vi "Main.vi"() -> ()   [LabVIEW 2018]
panel:
  in  "Save":bool
  in  "Data":T1={"Name"="Kevin", "Depart"="¦Û°Ê¤Æ±±¨î³¡", "Company"="¸s²Ý¯à·½ªÑ¥÷¦³­­¤½¥q", "E-Mail"="egdep33@hephasenergy.com", "Extension"="213", "Address"="·s¦Ë¿¤¶é°Ï¤G¸ô60¸¹1¼Ó"}
  in  "WebBrowser":refnum<k7>(container)
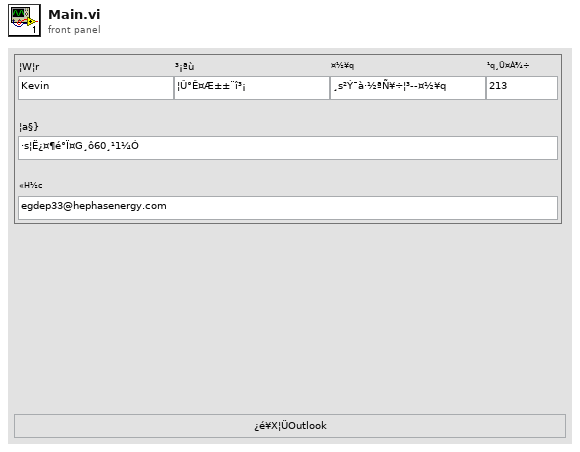
[diagram p1: front panel]
types:
  T1 = cluster{"Name":string, "Depart":string, "Company":string, "E-Mail":string, "Extension":string, "Address":string}
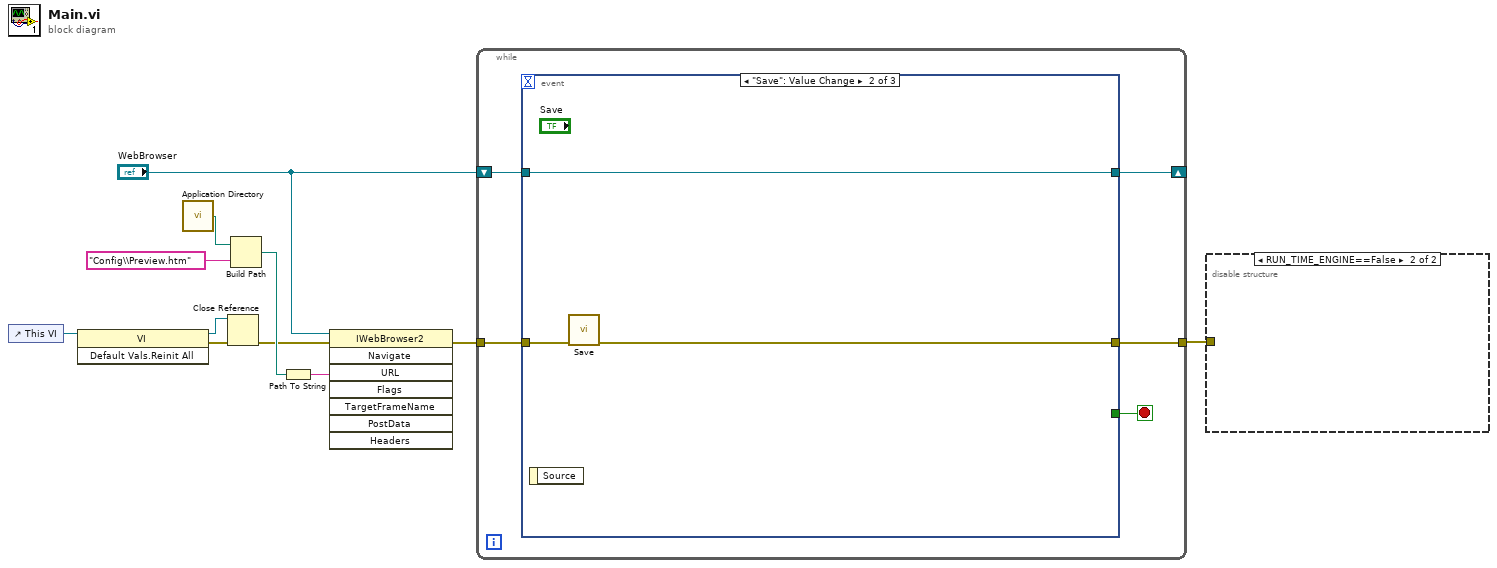
[diagram p0: block diagram]
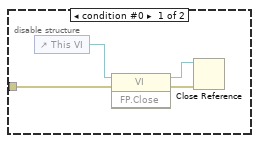
[diagram p2: hidden frame]
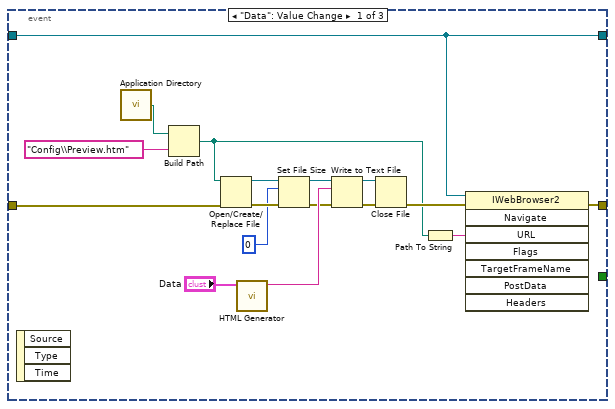
[diagram p3: hidden frame]
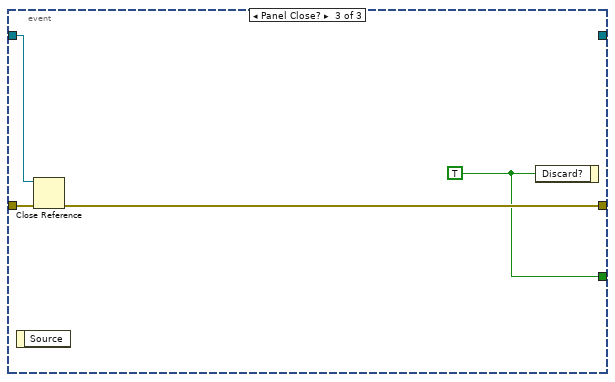
[diagram p4: hidden frame]
diagram:
  n1 = control-ref of="This VI"() -> (w5:refnum<vi>)
  n2 = invoke class="VI" method="Default Vals.Reinit All"(reference=w5) -> (reference out=w3:refnum<vi>, error out=w4:errorcluster)  [unwired: 2 in, 1 out]
  n3 = call <vilib>:"Application Directory.vi"() -> ("Application Directory"=w11:path)
  n4 = Close Reference(reference=w3, error in (no error)=w4) -> (error out=w2:errorcluster)
  n5 = Build Path(base path=w11, name or relative path="Config\\Preview.htm") -> (appended path=w8:path)
  n6 = Path To String(path=w8) -> (string=w9:string)
  n7 = invoke class="IWebBrowser2" method="Navigate"(reference="WebBrowser", error in=w2, "URL"=w9) -> (error out=w7:errorcluster)  [unwired: 5 in, 7 out]
  n8 = while {
    tunnel: w7 -> [w16]
    shift-right: [w13] -> _
    shift-left: "WebBrowser" -> [w15]
    tunnel: [w14] -> w1
    stop <- w12 stop-if-true
    n9 = event shown="[1] \"Save\": Value Change" {
      selector: _ -> [_ _ _]
      dyn-events: _ -> [_ _ _]
      timeout: _ -> [_ _ _]
      tunnel: w16 -> [w23 w35 w40]
      tunnel: w15 -> [w24 w36 w39]
      tunnel: [w25 w34 w38] -> w14
      tunnel: [w24 w36 _] -> w13
      tunnel: [_ _ w37] -> w12
      event "Data": Value Change {
        n10 = event-data() -> ()  [unwired: 1 in, 3 out]
        n11 = call <vilib>:"Application Directory.vi"() -> ("Application Directory"=w32:path)
        n12 = Build Path(base path=w32, name or relative path="Config\\Preview.htm") -> (appended path=w26:path)
        n13 = Open/Create/Replace File(file path (use dialog)=w26, error in=w23) -> (refnum out=w21:refnum<file>, error out=w20:errorcluster)  [unwired: 4 in, 1 out]
        n14 = call "HTML Generator.vi"("Data"="Data") -> ("HTML Out"=w29:string)  [unwired: 10 in]
        n15 = Set File Size(4:w20, 6:i64 0 ("size (in bytes)"), 7:w21) -> (0:w19:errorcluster, 3:w18:refnum<file>)
        n16 = Write to Text File(file (use dialog)=w18, text=w29, error in=w19) -> (refnum out=w31:refnum<file>, error out=w33:errorcluster)  [unwired: 1 in, 1 out]
        n17 = Close File(refnum=w31, error in=w33) -> (error out=w28:errorcluster)  [unwired: 1 out]
        n18 = Path To String(path=w26) -> (string=w27:string)
        n19 = invoke class="IWebBrowser2" method="Navigate"(reference=w24, error in=w28, "URL"=w27) -> (error out=w25:errorcluster)  [unwired: 5 in, 7 out]
      }
      event "Save": Value Change {
        n20 = event-data() -> ()  [unwired: 1 in, 1 out]
        n21 = call "Save.vi"("error in (no error)"=w35) -> ("error out"=w34:errorcluster)  [unwired: 10 in]
      }
      event Panel Close? {
        w37 = TRUE
        n22 = event-data() -> ()  [unwired: 1 in, 1 out]
        n23 = Close Reference(reference=w39, error in (no error)=w40) -> (error out=w38:errorcluster)
        n24 = event-data("Discard?"=w37) -> ()  [unwired: 1 in, 1 out]
      }
    }
  }
  n25 = disable-structure shown="RUN_TIME_ENGINE==False" {
    disable-tunnel: w1 -> [w42 _]
    frame condition #0 {
      n26 = control-ref of="This VI"() -> (w41:refnum<vi>)
      n27 = invoke class="VI" method="FP.Close"(reference=w41, error in=w42) -> (reference out=w44:refnum<vi>, error out=w43:errorcluster)  [unwired: 1 in, 1 out]
      n28 = Close Reference(reference=w44, error in (no error)=w43) -> ()  [unwired: 1 out]
    }
    frame condition #1 (active) {
    }
  }
